vi "Index Array.vi"(8 "error in (no error)":errorcluster, 9 "Index in":i32, 11 "Config Element in":refnum<class "Config Element.lvclass">) -> (0 "error out":errorcluster, 1 "Element":refnum<class "Config Element.lvclass">, 3 "Config Element out":refnum<class "Config Element.lvclass">)   [LabVIEW 2020, in "CDM-Config.lvlib" / "Config Element.lvclass"]
uses:
  Config Element.lvclass
  Config Element.lvclass/Config Element.ctl
  Config Manager/Config Manager.lvclass
  Value Type.ctl
  CDM-Config.lvlib
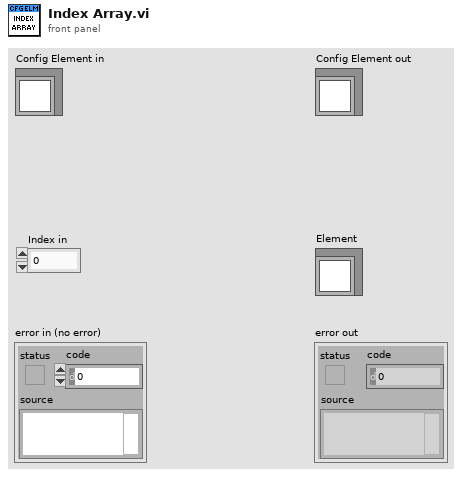
[diagram p1: front panel]
types:
  T1 = typedef "CDM-Config.lvlib/Value Type.ctl" = enum16{"String", "Number", "Bool", "Object", "Array"}
  T2 = typedef "CDM-Config.lvlib/Config Element.lvclass/Ref Data.ctl" = cluster{"Node Info":T3, "Owner":refnum<class>, "Changed":bool, "Name":string, "Meta Data":T4[], "Value Type":T1, "Value":variant}
  T3 = typedef "CDM-Config.lvlib/Node Info.ctl" = cluster{"Index":i32, "Parent":i32, "Children":i32[]}
  T4 = typedef "CDM-Config.lvlib/Meta Data.ctl" = cluster{"Name":string, "Value":string}
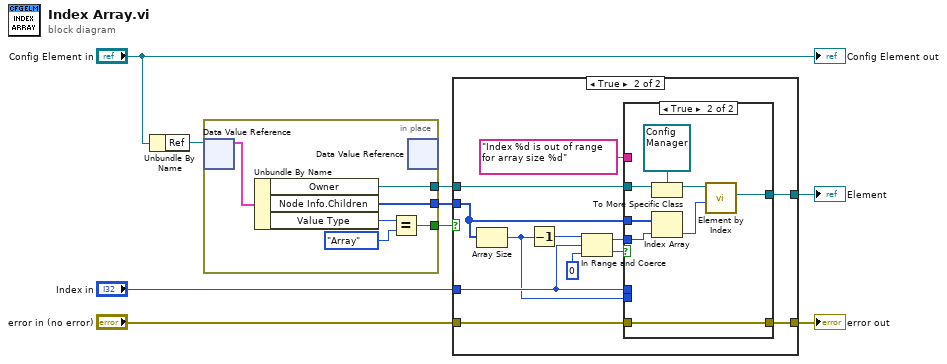
[diagram p0: block diagram]
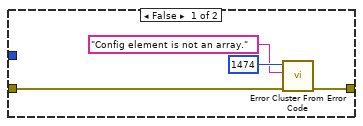
[diagram p2: hidden frame]
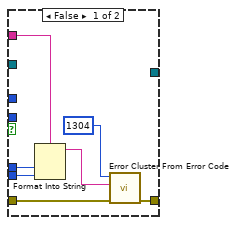
[diagram p3: hidden frame]
diagram:
  n1 = Unbundle By Name("Config Element in") -> ("Ref"=w9:refnum<data-value>)
  n2 = in-place {
    in-place-border: [w14] -> w7
    in-place-border: [w10] -> w5
    in-place-border: [w13] -> w6
    n3 = in-place-dvr #1(w9) -> (w15:T2)  [unwired: 1 out]
    n4 = Unbundle By Name(w15) -> ("Owner"=w13:refnum<class>, "Node Info.Children"=w14:i32[], "Value Type"=w12:T1)
    n5 = Equal?(x=w12, y=Value_Type."Array") -> (x = y?=w10:bool)
    n6 = in-place-dvr #1() -> ()  [unwired: 1 in, 2 out]
  }
  n7 = case shown="True" w5 {
    tunnel: w7 -> [_ w29]
    tunnel: w6 -> [_ w31]
    tunnel: "Index in" -> [_ w22]
    tunnel: [_ w30] -> w3
    tunnel: [w19 w24] -> w2
    tunnel: "error in (no error)" -> [w18 w23]
    frame False {
      n8 = call <vilib>:"Error Cluster From Error Code.vi"("error in (no error)"=w18, "error message (\"\")"="Config element is not an array.", "error code (0)"=1474) -> ("error out"=w19:errorcluster)  [unwired: 6 in]
    }
    frame True {
      n9 = Array Size(array=w29) -> (size(s)=w20:i32)
      n10 = Decrement(x=w20) -> (x-1=w26:i32)
      n11 = In Range and Coerce(upper limit=w26, x=w22, lower limit=0) -> (coerced(x)=w27:i32, In Range?=w25:bool)
      n12 = case shown="True" w25 {
        tunnel: w31 -> [_ w46]
        tunnel: [_ w42] -> w30
        tunnel: w29 -> [_ w41]
        tunnel: w27 -> [_ w40]
        tunnel: [w38 w39] -> w24
        tunnel: w23 -> [w37 w39]
        tunnel: w22 -> [w36 _]
        tunnel: "Index %d is out of range for array size %d" -> [w35 _]
        tunnel: w20 -> [w34 _]
        frame False {
          n13 = Format Into String(format string=w35, w36, w34) -> (resulting string=w33:string)  [unwired: 2 in, 1 out]
          n14 = call <vilib>:"Error Cluster From Error Code.vi"("error in (no error)"=w37, "error message (\"\")"=w33, "error code (0)"=1304) -> ("error out"=w38:errorcluster)  [unwired: 6 in]
        }
        frame True {
          n15 = To More Specific Class(target class=refnum<class "Config Manager.lvclass"> refnum ("CDM-Config.lvlib:Config Manager.lvclass"), reference=w46) -> (specific class reference=w44:refnum<class "Config Manager.lvclass">)  [unwired: 1 in, 1 out]
          n16 = Index Array(array=w41, index=w40) -> (element=w43:i32)
          n17 = call "Element by Index.vi"("Index"=w43, "Config Manager in"=w44) -> ("Element"=w42:refnum<class "Config Element.lvclass">)  [unwired: 7 in, 2 out]
        }
      }
    }
  }
  "error out" <- w2
  "Element" <- w3
  "Config Element out" <- "Config Element in"
